vi "DriveDirection.vi"() -> ()   [LabVIEW 2016]
uses:
  Refname/Motors.ctl
  Refname/Refname to String (Motors).vi
  <vilib>/addons/control/pid/pid.llb/PID (DBL).vi
  <vilib>/addons/control/pid/NI_PID_pid.lvlib
panel:
  out "Error out":errorcluster
  in  "Position Desired":dbl format="%#_13g"
  in  "Wheel Power":dbl format="%#_13g"
  in  "error constant":errorcluster
  in  "Tolerance":dbl format="%#_13g"
  in  "output range":cluster{"output high":dbl, "output low":dbl}={"output high"=100.0, "output low"=-100.0}
  in  "PID gains":T1={"proportional gain (Kc)"=1.0, "integral time (Ti, min)"=0.01, "derivative time (Td, min)"=0.0} {"derivative time (Td, min)" format="%.3f"; "integral time (Ti, min)" format="%.3f"; "proportional gain (Kc)" format="%.3f"}
  in  "Setpoint":dbl format="%#_13g"
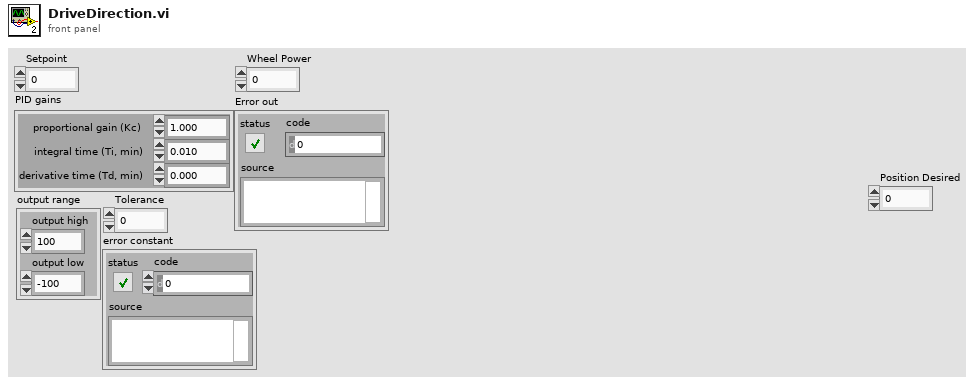
[diagram p1: front panel]
types:
  T1 = cluster{"proportional gain (Kc)":dbl, "integral time (Ti, min)":dbl, "derivative time (Td, min)":dbl}
  T2 = typedef "Motors.ctl" = enum16{"Wheel 1", "Swerve 1", "Wheel 2", "Swerve 2", "Wheel 3", "Swerve 3", "Wheel 4", "Swerve 4"}
  T3 = typedef "WPI_MotorControlDeviceRef.ctl" = cluster{"DeviceStatus":errorcluster, "Type":T4, "PWM":cluster{"PWM Channel":T5, "DeadBand":T6}, "CAN":cluster{"Device Number":u8, "SetOutput VI Ref":variant, "GetOutput VI Ref":variant, "Enable VI Ref":variant, "Disable VI Ref":variant, "Data":variant}, "Invert":bool}
  T4 = typedef "WPI_MotorControlType.ctl" = enum16{"PWM", "CAN"}
  T5 = typedef "FPGA_DIOPWMChannel.ctl" = enum8{"PWM 0", "PWM 1", "PWM 2", "PWM 3", "PWM 4", "PWM 5", "PWM 6", "PWM 7", "PWM 8", "PWM 9", "PWM MXP 0", "PWM MXP 1", "PWM MXP 2", "PWM MXP 3", "PWM MXP 4", "PWM MXP 5", "PWM MXP 6", "PWM MXP 7", "PWM MXP 8", "PWM MXP 9", "Invalid"}
  T6 = typedef "WPI_PWMDeadband.ctl" = cluster{"Name":string, "maxPositivePwm":i32, "minPositivePwm":i32, "centerPwm":i32, "maxNegativePwm":i32, "minNegativePwm":i32, "angularRange":u16}
  T7 = typedef "WPI_CANTalonSRX_GlobalStatus.ctl" = cluster{"Applied Throttle":dbl, "Module Enabled":bool, "CAN Error":errorcluster, "Closed Loop Error":dbl, "Forward Limit Switch Closed":bool, "Reverse Limit Switch Closed":bool, "Sensor Position":dbl, "Sensor Velocity":dbl, "Current":dbl, "Sticky Fault - Over Temp":bool, "Sticky Fault - Under Voltage":bool, "Sticky Fault - Forward Limit":bool, "Sticky Fault - Reverse Limit":bool, "Sticky Fault - Forward Soft Limit":bool, "Sticky Fault - Reverse Soft Limit":bool, "Brake is Enabled":bool, "Encoder Position":dbl, "Encoder Velocity":dbl, "Encoder Index Count":dbl, "Encoder A Pin State":bool, "Encoder B Pin State":bool, "Encoder Index Pin State":bool, "Analog In":dbl, "Analog In Velocity":dbl, "Temperature (C)":dbl, "Battery Voltage":dbl, "Control 5 Is Supported":bool, "Current Profile Slot Select":dbl, "Pos Div 8":bool, "Vel Div 4":bool, "Pulse Width Position":i32, "Pulse Width Velocity":i32, "Pulse Width Rise To Rise (us)":i32, "Pulse Width Rise To Fall (us)":i32, "Mot Prof Active Is Under Run":bool, "Mot Prof Active Has Under Run":bool, "Mot Prof Active Is Last":bool, "Mot Prof Active Velocity Only":bool, "Mot Prof Active Is Valid":bool, "Mot Prof Buffer Is Full":bool, "Mot Prof Active Profile Slot Select":i32, "Mot Prof NextID":i32, "Mot Prof Count":i32, "Mot Prof Active Velocity":dbl, "Mot Prof Active Position":dbl, "Mot Prof Output Enable":i32}
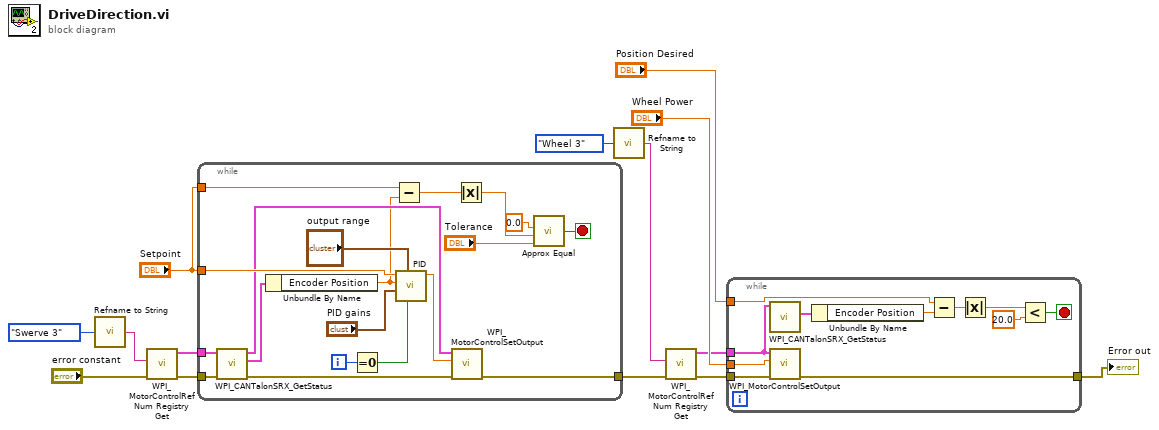
[diagram p0: block diagram]
diagram:
  n1 = call-poly "Refname to String.vi"("Enum"=Motors."Swerve 3") -> ("String"=w13:string)
  n2 = call <vilib>:"WPI_MotorControlRefNum Registry Get.vi"("error in (no error)"="error constant", "refnum name"=w13) -> ("error out"=w9:errorcluster, "MotorControlDevRef"=w12:T3)  [unwired: 8 in]
  n3 = while {
    tunnel: w12 -> [w33]
    tunnel: "Setpoint" -> [w31]
    tunnel: "Setpoint" -> [w19]
    tunnel: w9 -> [w17]
    tunnel: [w15] -> w5
    i -> [w28]
    stop <- w23 stop-if-true
    n4 = call <vilib>:"WPI_CANTalonSRX_GetStatus.vi"("error in (no error)"=w17, "CAN Talon SRX Ref"=w33) -> ("error out"=w16:errorcluster, "Talon SRX Status"=w32:T7, "CAN Talon SRX Ref"=w25:T3)  [unwired: 7 in]
    n5 = Unbundle By Name(w32) -> ("Encoder Position"=w18:dbl)
    n6 = Equal To 0?(x=w28) -> (x = 0?=w27:bool)
    n7 = Subtract(x=w19, y=w18) -> (x-y=w20:dbl)
    n8 = call-poly <vilib>:"PID.vi"("reinitialize? (F)"=w27, "output range"="output range", "PID gains"="PID gains", "process variable"=w18, "setpoint"=w31) -> ("output"=w26:dbl)  [unwired: 5 in, 1 out]
    n9 = call <vilib>:"WPI_MotorControlSetOutput.vi"("error in (no error)"=w16, "Output"=w26, "MotorControlDevRef"=w25) -> ("error out"=w15:errorcluster)  [unwired: 6 in, 2 out]
    n10 = Absolute Value(x=w20) -> (abs(x)=w21:dbl)
    n11 = call "Approx Equal.vi"("Tolerance"="Tolerance", "b"=w21, "a"=0.0) -> ("a == b?"=w23:bool)  [unwired: 1 in]
  }
  n12 = call-poly "Refname to String.vi"("Enum"=Motors."Wheel 3") -> ("String"=w7:string)
  n13 = call <vilib>:"WPI_MotorControlRefNum Registry Get.vi"("error in (no error)"=w5, "refnum name"=w7) -> ("error out"=w4:errorcluster, "MotorControlDevRef"=w2:T3)  [unwired: 8 in]
  n14 = while {
    tunnel: "Wheel Power" -> [w44]
    tunnel: w2 -> [w42]
    tunnel: w4 -> [w43]
    tunnel: "Position Desired" -> [w37]
    tunnel: [w34] -> w1
    stop <- w40 stop-if-true
    n15 = call <vilib>:"WPI_CANTalonSRX_GetStatus.vi"("CAN Talon SRX Ref"=w42) -> ("Talon SRX Status"=w41:T7)  [unwired: 8 in, 2 out]
    n16 = call <vilib>:"WPI_MotorControlSetOutput.vi"("error in (no error)"=w43, "Output"=w44, "MotorControlDevRef"=w42) -> ("error out"=w34:errorcluster)  [unwired: 6 in, 2 out]
    n17 = Unbundle By Name(w41) -> ("Encoder Position"=w38:dbl)
    n18 = Subtract(x=w37, y=w38) -> (x-y=w36:dbl)
    n19 = Absolute Value(x=w36) -> (abs(x)=w35:dbl)
    n20 = Less?(x=w35, y=20.0) -> (x < y?=w40:bool)
  }
  "Error out" <- w1
